vi "AVS_Done.vi"() -> (17 "Output Value":i32)   [LabVIEW 2013, in "AvaSpec.lvlib" / "Avantes Spectrometer Functions.lvlib"]
uses:
  Avantes Spectrometer Functions.lvlib
  AS5216.dll
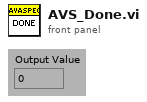
[diagram p1: front panel]
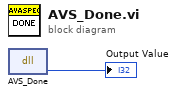
[diagram p0: block diagram]
diagram:
  n1 = dll-call lib="C:/Users/dhstuart/Dropbox/CLTC/avantesSpectrometer/Libraries/AS-5216-DLL/polling_mc/AS5216.dll" fn="AVS_Done"() -> (→"Output Value":i32)  [unwired: 3 in, 2 out]
